vi "test1-TestModuleStatusVI.vi"(8 "error in (no error)":errorcluster, 11 "TestCase in":refnum<class "testcase-CSMManagementAPI.lvclass">) -> (0 "error out":errorcluster, 3 "TestCase out":refnum<class "testcase-CSMManagementAPI.lvclass">)   [LabVIEW 2017, in "testcase-CSMManagementAPI.lvclass"]
uses:
  testcase-CSMManagementAPI.lvclass
  src/user.lib/_NEVSTOP/Communicable State Machine(CSM)/_Support/Typedef/_CSM_MODE.ctl
  src/user.lib/_NEVSTOP/Communicable State Machine(CSM)/AdvanceAPI/CSM - Revert Arguments-Safe String.vi
  src/user.lib/_NEVSTOP/Communicable State Machine(CSM)/_Shared/Trim Single-line Text.vi
  src/user.lib/_NEVSTOP/Communicable State Machine(CSM)/AdvanceAPI/CSM - Make String Arguments Safe.vi
  src/user.lib/_NEVSTOP/Communicable State Machine(CSM)/AdvanceAPI/CSM - Break Down Multiple States String.vi
  src/user.lib/_NEVSTOP/Communicable State Machine(CSM)/AdvanceAPI/CSM - Compact Multiple States.vi
  src/user.lib/_NEVSTOP/Communicable State Machine(CSM)/AdvanceAPI/CSM - Keywords.vi
  <vilib>/addons/_JKI Toolkits/VI Tester/TestCase.llb/TestCase.lvclass
  src/user.lib/_NEVSTOP/Communicable State Machine(CSM)/Communicable State Machine.lvlib
  src/user.lib/_NEVSTOP/Communicable State Machine(CSM)/_Support/Typedef/_CSM_List Module Scope.ctl
  C:/Program Files (x86)/National Instruments/LabVIEW 2017/vi.lib/addons/_JKI Toolkits/VI Tester/TestCase.llb/TestCase.lvclass
panel:
  out "State History":string
  out "LoopCount":i32
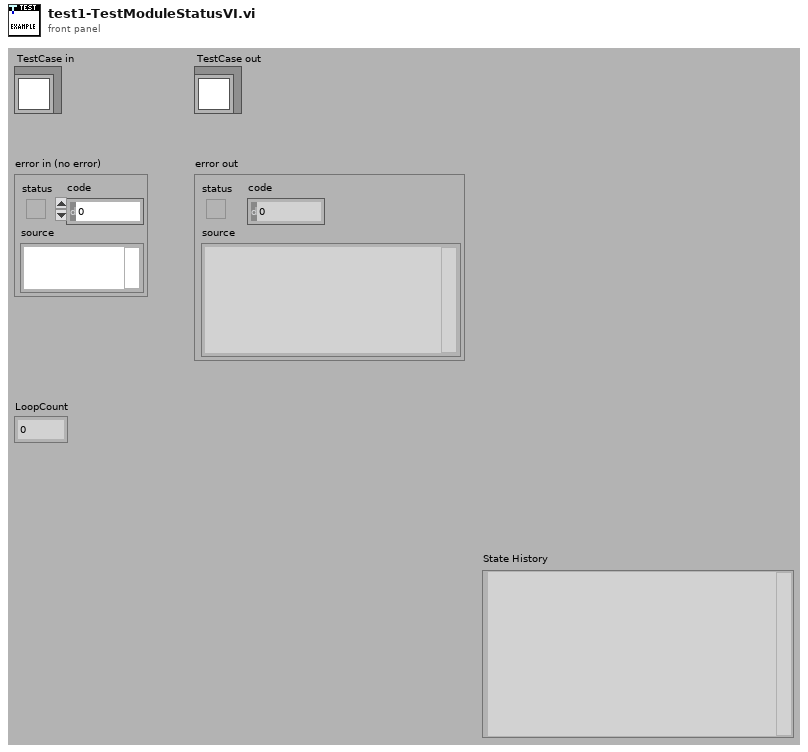
[diagram p1: front panel]
types:
  T1 = typedef "Communicable State Machine.lvlib/_CSM_MODE.ctl" = enum16{"Not Exist", "Stand Alone", "CSM", "Worker", "Worker Agent", "Chain Node", "Chain"}
  T2 = cluster{"CSM Name (Dup)":string, "Mode":T1, "#Nodes":i32}[]
  T3 = typedef "Communicable State Machine.lvlib/_CSM_List Module Scope.ctl" = enum16{"Normal", "System Only", "All"}
  T4 = enum32{"Invalid", "Standard", "Closed", "Hidden", "Minimized", "Maximized"}
  T5 = enum32{"invalid app kind", "Development System", "Run Time System", "Student Edition", "Embedded LabVIEW", "Evaluation", "Custom"}
  T6 = typedef "Communicable State Machine.lvlib/_CSM_Response Source Message.ctl" = cluster{"‘State":string, "’Arguments":string, "’Error":errorcluster}
  T7 = cluster{"Current VI Reference":refnum<vi>, "Close Panel on Exit?":bool}
  T8 = cluster{"Core":cluster{"Current VI Reference":refnum<vi>, "Close Panel on Exit?":bool}, "Your Boolean data":bool, "Your string data":string, "Module Status":cluster{"CSM Name (Dup)":string, "Mode":T1, "#Nodes":i32}}
  T9 = cluster{"CSM Name (Dup)":string, "Mode":T1, "#Nodes":i32}
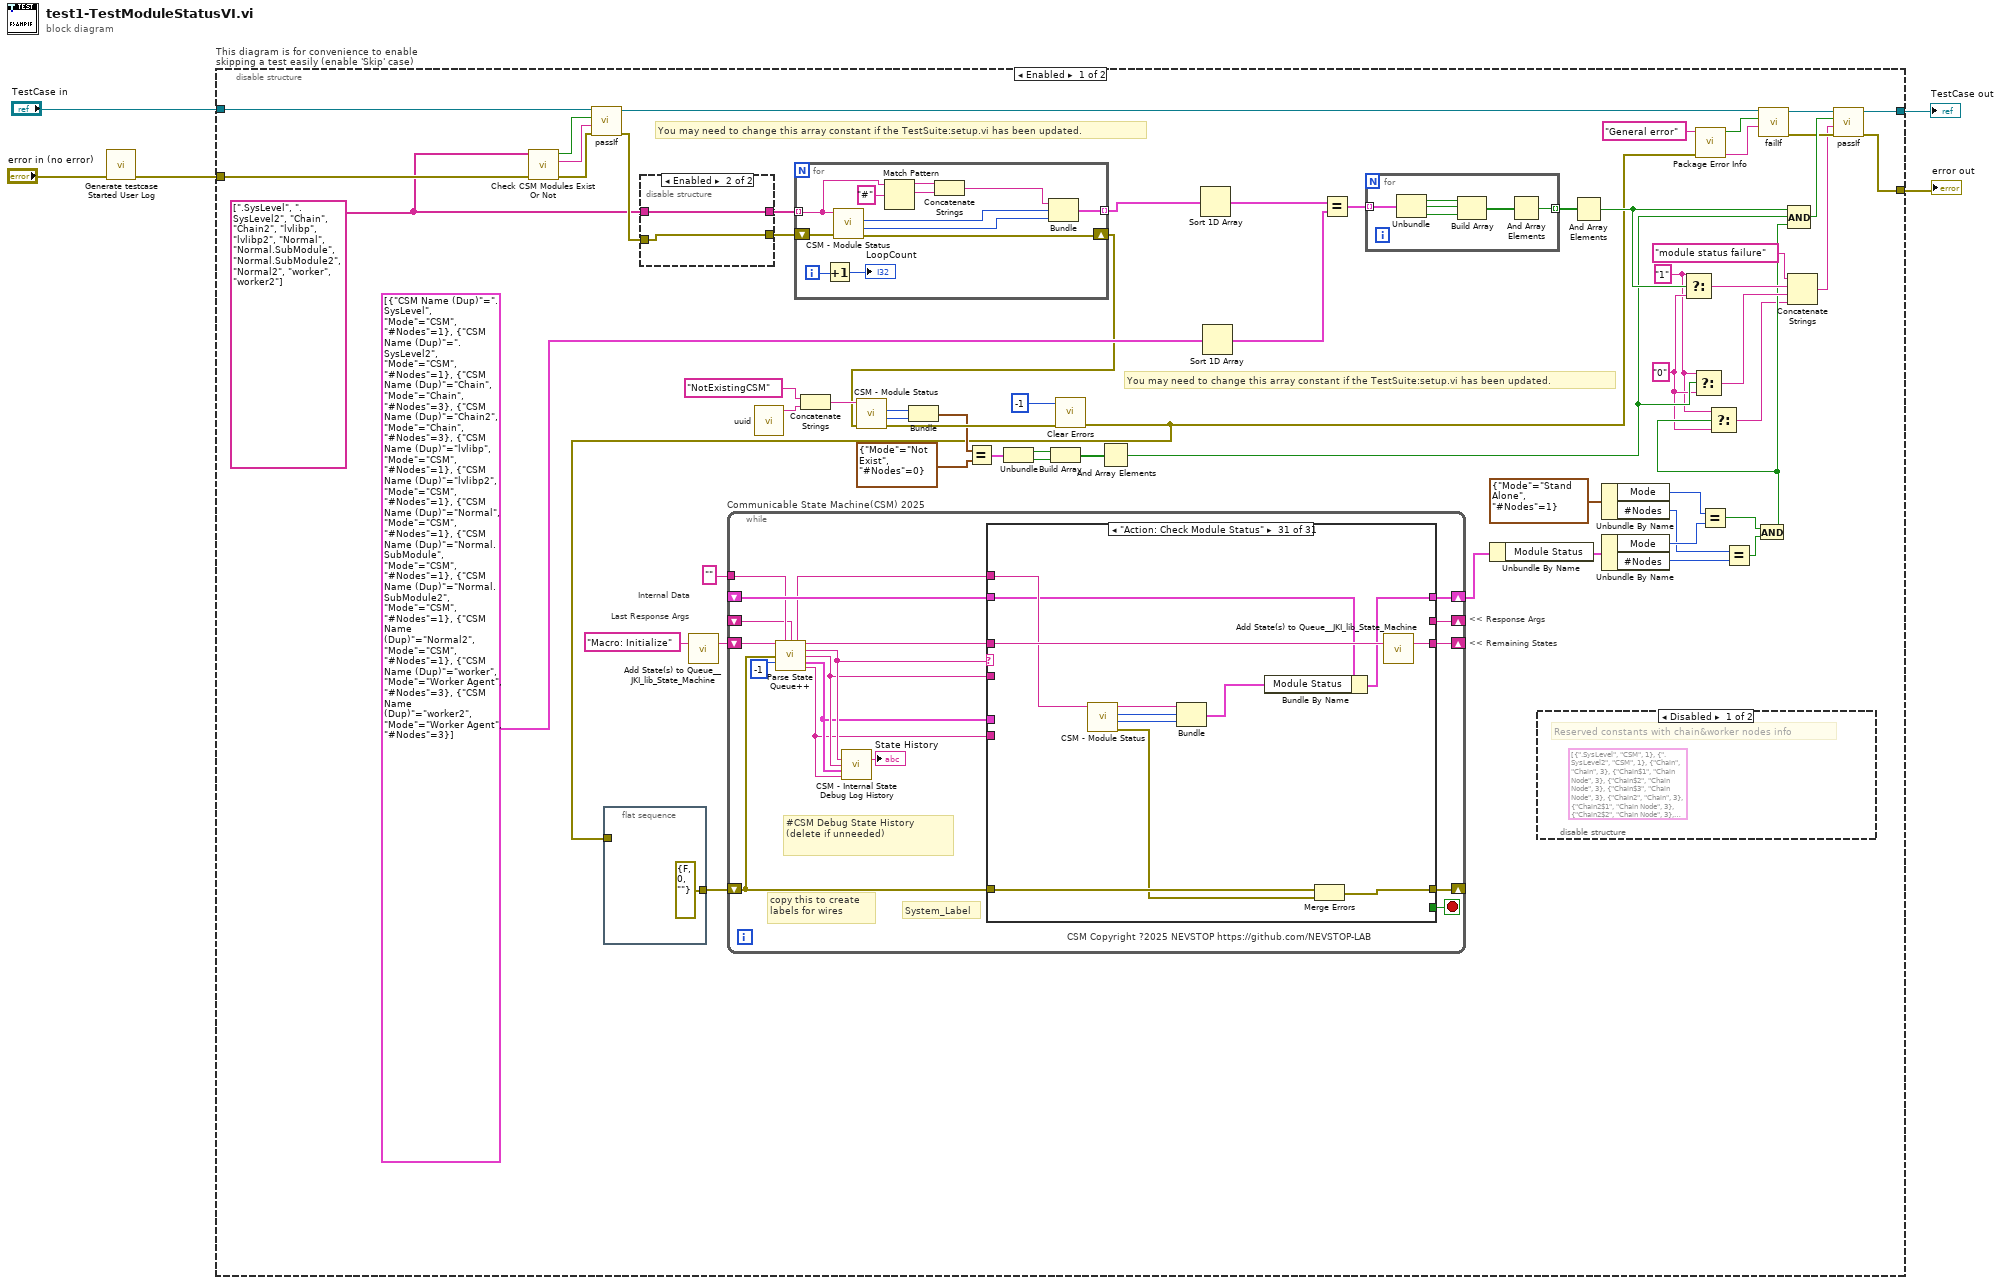
[diagram p0: block diagram]
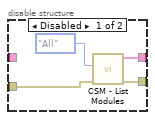
[diagram p3: hidden frame]
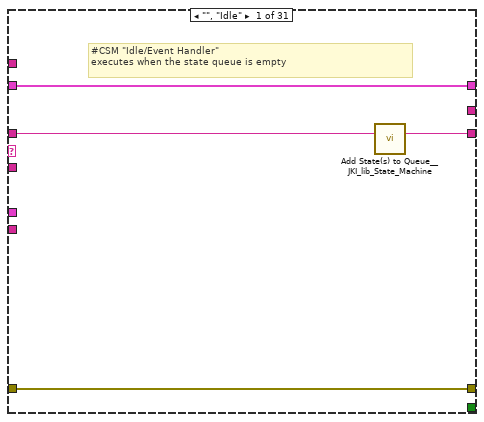
[diagram p4: hidden frame]
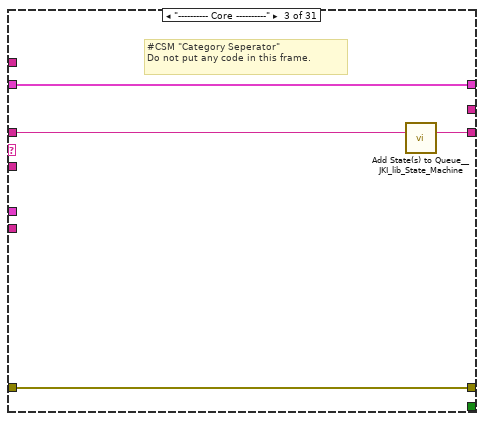
[diagram p6: hidden frame]
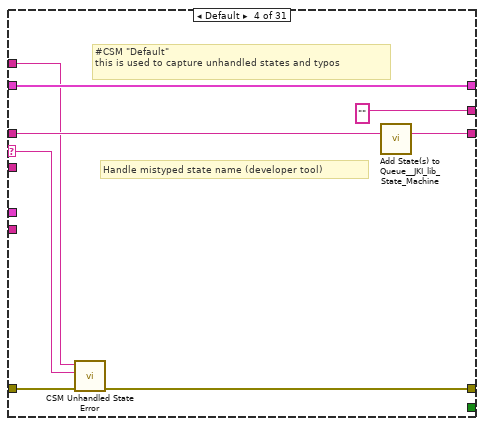
[diagram p7: hidden frame]
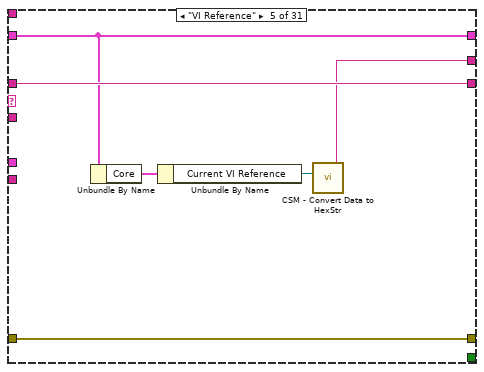
[diagram p8: hidden frame]
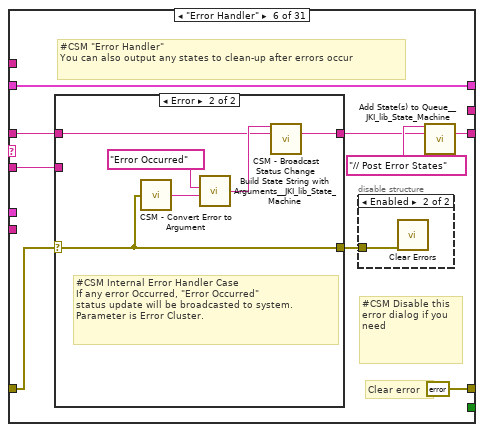
[diagram p9: hidden frame]
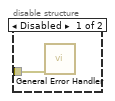
[diagram p10: hidden frame]
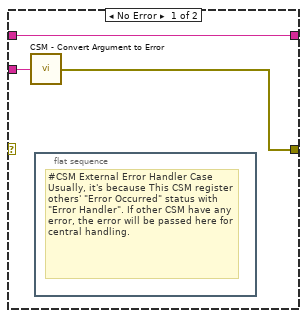
[diagram p11: hidden frame]
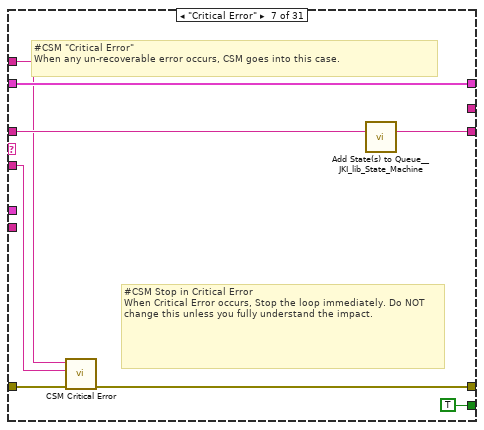
[diagram p12: hidden frame]
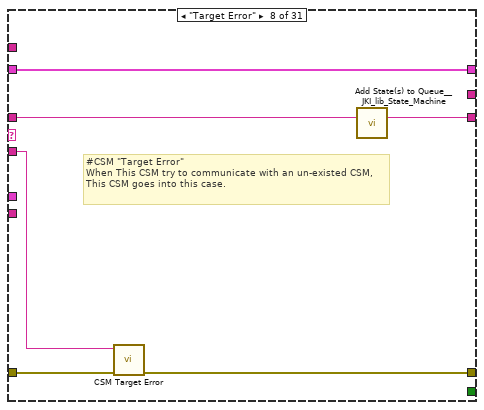
[diagram p13: hidden frame]
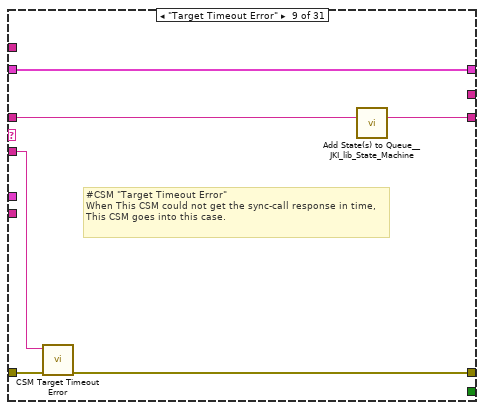
[diagram p14: hidden frame]
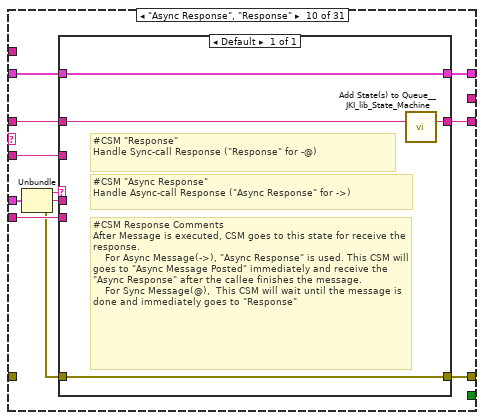
[diagram p15: hidden frame]
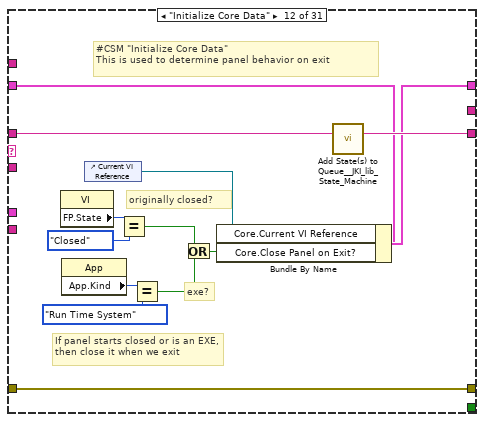
[diagram p17: hidden frame]
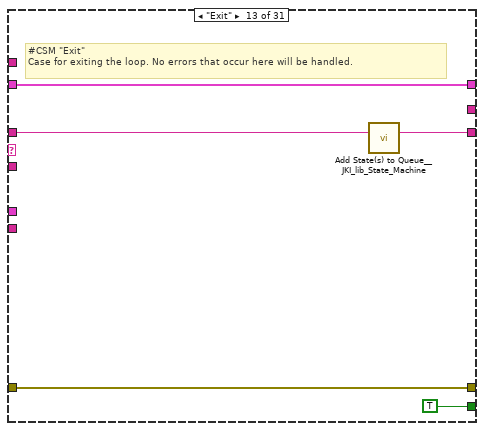
[diagram p18: hidden frame]
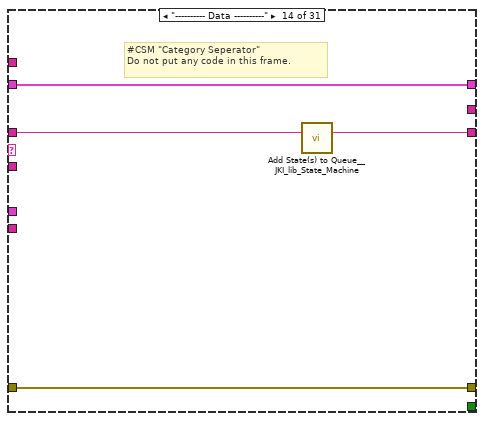
[diagram p19: hidden frame]
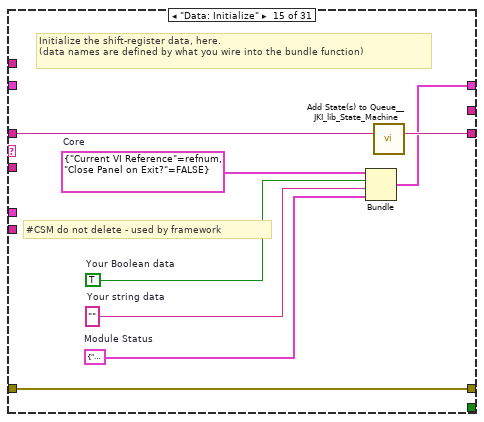
[diagram p20: hidden frame]
diagram:
  n1 = call "Generate testcase Started User Log.vi"("Error In"="error in (no error)") -> ("error out"=w1:errorcluster)  [unwired: 10 in]
  n2 = disable-structure "This diagram is for convenience to enable skipping a test easily (enable 'Skip' case)" shown="Enabled" {
    disable-tunnel: "TestCase in" -> [w27 w384]
    disable-tunnel: [w65 w382] -> w2
    disable-tunnel: [w64 w383] -> w4
    disable-tunnel: w1 -> [w26 w381]
    frame Enabled {
      w12 = "0" ("f")
      w11 = "1"
      w6 = string[] [".SysLevel", ".SysLevel2", "Chain", "Chain2", "lvlibp", "lvlibp2", "Normal", "Normal.SubModule", "Normal.SubModule2", "Normal2", "worker", "worker2"] ("Module Names in All Scope")
      # "You may need to change this array constant if the TestSuite:setup.vi has been updated."
      # "You may need to change this array constant if the TestSuite:setup.vi has been updated."
      # "Last Response Args"
      # "Internal Data"
      # "<< Response Args"
      # "<< Remaining States"
      n3 = call "Check CSM Modules Exist Or Not.vi"("error in"=w26, "CSM names in"=w6) -> ("error out"=w28:errorcluster, "Debug string"=w29:string, "All Modules Exist?"=w30:bool)  [unwired: 7 in]
      n4 = call-dynamic "passIf.vi"("error in (no error)"=w28, "message (\"\")"=w29, "pass"=w30, "TestCase in"=w27) -> ("error out"=w25:errorcluster, "TestCase out"=w22:refnum<class "testcase-CSMManagementAPI.lvclass">)  [unwired: 6 in]
      n5 = flat-sequence {
        tunnel: [errorcluster {"status"=FALSE, "code"=0, "source"=""} ("error out")] -> w63
        tunnel: w7 -> [_]
        frame #0 {
        }
      }
      n6 = disable-structure shown="Enabled" {
        disable-tunnel: [w70 w73] -> w67
        disable-tunnel: [w69 w72] -> w66
        disable-tunnel: w25 -> [w68 w73]
        disable-tunnel: w6 -> [_ w72]
        frame Disabled {
          n7 = call "CSM - List Modules.vi"("Error In"=w68, "Scope (Normal)"=_CSM_List_Module_Scope."All") -> ("error out"=w70:errorcluster, "Module Names"=w69:string[])  [unwired: 8 in]
        }
        frame Enabled {
        }
      }
      n8 = call <vilib>:"Add State(s) to Queue__JKI_lib_State_Machine.vi"("State(s) in (\"\")"="Macro: Initialize" ("Init State(\"Macro: Initialize\")")) -> ("States Out"=w60:string)  [unwired: 14 in]
      n9 = while "Communicable State Machine(CSM) 2025" {
        shift-right: [w93] -> w59
        shift-left: _ -> [w92]
        shift-right: [w96] -> _
        shift-left: w63 -> [w91]
        shift-right: [w95] -> _
        shift-left: w60 -> [w97]
        tunnel: "" ("Name (\"\" to Use UUID)") -> [w89]
        shift-right: [w90] -> _
        shift-left: _ -> [w83]
        stop <- w94 stop-if-true
        # "#CSM Debug State History\n(delete if unneeded)"
        # "copy this to create labels for wires"
        # "System_Label"
        # "CSM Copyright ?2025 NEVSTOP https://github.com/NEVSTOP-LAB"
        n10 = call "Parse State Queue++.vi"("State Queue"=w97, "Name (\"\" to Use UUID)"=w89, "Response Arguments"=w83, "Previous Error"=w91, "Dequeue (1 ms)"=-1 ("Timeout")) -> ("Name Used"=w84:string, "Remaining States"=w98:string, "Current State"=w88:string, "Arguments"=w87:string, "Additional Information"=w86:T6, "Source CSM"=w85:string)  [unwired: 5 in]
        n11 = call "CSM - Internal State Debug Log History.vi"("State"=w88, "Arguments (\"\")"=w87, ">> Response Source Message >>"=w86, "Source (\"\")"=w85) -> ("Debug Log"=→"State History":string)  [unwired: 11 in]
        n12 = case shown="\"Action: Check Module Status\"" w88 {
          selector: w88 -> [_ _ _ w112 _ _ _ _ _ _ _ _ _ _ _ _ _ _ _ _ _ _ _ _ _ _ _ _ _ _ _]
          tunnel: w98 -> [w99 w104 w109 w116 w122 w128 w149 w155 w161 w169 w180 w194 w199 w203 w211 w213 w220 w224 w228 w234 w249 w318 w323 w330 w332 w336 w341 w348 w352 w356 w368]
          tunnel: w87 -> [_ _ _ _ _ w127 w145 w154 w159 w168 _ _ _ _ _ _ _ _ _ w229 w243 _ _ _ _ _ w339 _ _ _ _]
          tunnel: w92 -> [w100 w103 w106 w114 w121 w131 w150 w156 w162 w171 w179 w187 w197 w200 _ w212 w215 w221 w226 w232 w245 w315 w320 w327 w331 w335 w340 w345 w349 w353 w361]
          tunnel: [w101 w105 w107 w110 w123 errorcluster {"status"=FALSE, "code"=0, "source"=""} ("error out") w146 w152 w158 w174 w181 w191 w196 w201 w208 w214 w216 w222 w225 w230 w246 w316 w321 w328 w333 w337 w342 w346 w350 w354 w358] -> w96
          tunnel: w91 -> [w101 w105 w107 w117 w123 w129 w151 w153 w160 _ w181 w191 w196 w201 w208 w214 w217 w222 w225 w231 w247 w316 w321 w328 w333 w337 w342 w346 w350 w354 w366]
          tunnel: [w102 w104 w108 w115 w122 w124 w148 w157 w163 w170 w180 w193 w198 w202 w210 w213 w219 w223 w227 w233 w248 w317 w322 w329 w332 w336 w341 w347 w351 w355 w367] -> w95
          tunnel: [_ _ _ _ _ _ TRUE _ _ _ _ _ TRUE _ _ _ _ _ _ _ _ _ _ _ _ _ _ _ _ _ _] -> w94
          tunnel: [w100 w103 w106 w114 w121 w131 w150 w156 w162 w172 w179 w192 w197 w200 w209 w212 w215 w221 w226 w232 w245 w315 w320 w327 w331 w335 w340 w345 w349 w353 w360] -> w93
          tunnel: w85 -> [_ _ _ _ _ _ _ _ _ w166 _ _ _ _ _ _ _ _ _ _ _ _ _ _ _ _ _ _ _ _ _]
          tunnel: w86 -> [_ _ _ _ _ _ _ _ _ w173 _ _ _ _ _ _ _ _ _ _ _ _ _ _ _ _ _ _ _ _ _]
          tunnel: [_ _ _ "" w118 _ _ _ _ _ _ _ _ _ _ _ _ _ _ _ _ _ _ _ _ "API1 Response" w338 _ _ _ _] -> w90
          tunnel: w84 -> [_ _ _ w111 _ _ w144 _ _ _ _ _ _ _ _ _ _ _ _ _ _ _ _ _ _ _ _ _ _ _ w365]
          frame "", "Idle" {
            # "#CSM \"Idle/Event Handler\"\nexecutes when the state queue is empty"
            n13 = call <vilib>:"Add State(s) to Queue__JKI_lib_State_Machine.vi"("State(s) in (\"\")"=w99) -> ("States Out"=w102:string)  [unwired: 14 in]
          }
          frame "CSM Documentation" {
            # "#CSM README FIRST\n\nCommunicable State Machine(CSM) is a LabVIEW application framework that builds upon JKI State Machine(JKISM). It follows the pattern of JKISM and extends the keywords to describe message communication between modules, including concepts such as Sync-Message, Async-Message, Subscription/Unsubscription of status - essential elements for creating reusable code modules. For more information, please visit the CSM wiki: https://nevstop-lab.github.io/CSM-Wiki/\n\nFor instructions on JKI State Machine, visit: http://jki.net/state-machine/\nFor information about CSM, visit: https://github.com/NEVSTOP-LAB"
            # "#CSM \"Documentation\"\nCase for holding CSM Documenation"
          }
          frame "---------- Core ----------" {
            # "#CSM \"Category Seperator\"\nDo not put any code in this frame."
            n14 = call <vilib>:"Add State(s) to Queue__JKI_lib_State_Machine.vi"("State(s) in (\"\")"=w109) -> ("States Out"=w108:string)  [unwired: 14 in]
          }
          frame Default {
            # "#CSM \"Default\"\nthis is used to capture unhandled states and typos"
            # "Handle mistyped state name (developer tool)"
            n15 = call "CSM Unhandled State Error.vi"("error in (no error)"=w117, "Undefined State"=w112, "CSM Name"=w111) -> ("error out"=w110:errorcluster)  [unwired: 8 in]
            n16 = call <vilib>:"Add State(s) to Queue__JKI_lib_State_Machine.vi"("State(s) in (\"\")"=w116) -> ("States Out"=w115:string)  [unwired: 14 in]
          }
          frame "VI Reference" {
            n17 = Unbundle By Name(w121) -> ("Core"=w120:T7)
            n18 = Unbundle By Name(w120) -> ("Current VI Reference"=w119:refnum<vi>)
            n19 = call "CSM - Convert Data to HexStr.vi"("Variant"=w119) -> ("HEX String (0-9,A-F)"=w118:string)  [unwired: 8 in]
          }
          frame "Error Handler" {
            # "#CSM Disable this error dialog if you need"
            # "#CSM \"Error Handler\"\nYou can also output any states to clean-up after errors occur"
            # "Clear error"
            n20 = case shown="Error" w129 {
              selector: w129 -> [_ w138]
              tunnel: [w137 w140] -> w125
              tunnel: w128 -> [w137 w139]
              tunnel: w127 -> [w136 _]
              tunnel: [w135 w138] -> w130
              frame No Error {
                n21 = call "CSM - Convert Argument to Error.vi"("Argument"=w136) -> ("Error"=w135:errorcluster)  [unwired: 4 in]
                n22 = flat-sequence {
                  frame #0 {
                    # "#CSM External Error Handler Case\nUsually, it's because This CSM register others' \"Error Occurred\" status with \"Error Handler\". If other CSM have any error, the error will be passed here for central handling."
                  }
                }
              }
              frame Error {
                # "#CSM Internal Error Handler Case \nIf any error Occurred, \"Error Occurred\" \nstatus update will be broadcasted to system.\nParameter is Error Cluster."
                n23 = call "CSM - Convert Error to Argument.vi"("Error"=w138) -> ("Argument"=w142:string)  [unwired: 4 in]
                n24 = call <vilib>:"Build State String with Arguments__JKI_lib_State_Machine.vi"("Arguments (\"\")"=w142, "State"="Error Occurred" ("Status with Arguments")) -> ("State with Arguments"=w141:string)  [unwired: 4 in]
                n25 = call "CSM - Broadcast Status Change.vi"("Status With Arguments"=w141, "State Queue"=w139) -> ("Remaining States"=w140:string)  [unwired: 13 in]
              }
            }
            n26 = disable-structure shown="Enabled" {
              disable-tunnel: w130 -> [w133 w134]
              frame Disabled {
                n27 = call <vilib>:"General Error Handler.vi"("error in (no error)"=w133) -> ()  [unwired: 10 in, 5 out]
              }
              frame Enabled {
                n28 = call <vilib>:"Clear Errors.vi"("error in (no error)"=w134) -> ()  [unwired: 5 in, 2 out]
              }
            }
            n29 = call <vilib>:"Add State(s) to Queue__JKI_lib_State_Machine.vi"("State(s) in Front (\"\")"="// Post Error States", "State(s) in (\"\")"=w125) -> ("States Out"=w124:string)  [unwired: 13 in]
          }
          frame "Critical Error" {
            # "#CSM Stop in Critical Error\nWhen Critical Error occurs, Stop the loop immediately. Do NOT change this unless you fully understand the impact."
            # "#CSM \"Critical Error\"\nWhen any un-recoverable error occurs, CSM goes into this case."
            n30 = call "CSM Critical Error.vi"("error in (no error)"=w151, "Arugments (As Reason)"=w145, "CSM Name"=w144) -> ("error out"=w146:errorcluster)  [unwired: 8 in]
            n31 = call <vilib>:"Add State(s) to Queue__JKI_lib_State_Machine.vi"("State(s) in (\"\")"=w149) -> ("States Out"=w148:string)  [unwired: 14 in]
          }
          frame "Target Error" {
            # "#CSM \"Target Error\"\nWhen This CSM try to communicate with an un-existed CSM, This CSM goes into this case."
            n32 = call "CSM Target Error.vi"("error in (no error)"=w153, "Arguments (As CSM Name)"=w154) -> ("error out"=w152:errorcluster)  [unwired: 9 in]
            n33 = call <vilib>:"Add State(s) to Queue__JKI_lib_State_Machine.vi"("State(s) in (\"\")"=w155) -> ("States Out"=w157:string)  [unwired: 14 in]
          }
          frame "Target Timeout Error" {
            # "#CSM \"Target Timeout Error\"\nWhen This CSM could not get the sync-call response in time, This CSM goes into this case."
            n34 = call "CSM Target Timeout Error.vi"("error in (no error)"=w160, "Arguments (As CSM Name)"=w159) -> ("error out"=w158:errorcluster)  [unwired: 9 in]
            n35 = call <vilib>:"Add State(s) to Queue__JKI_lib_State_Machine.vi"("State(s) in (\"\")"=w161) -> ("States Out"=w163:string)  [unwired: 14 in]
          }
          frame "Async Response", "Response" {
            n36 = Unbundle(w173) -> ("‘State"=w167:string, "’Arguments"=w165:string, "’Error"=w164:errorcluster)
            n37 = case shown="Default" w167 {
              tunnel: [w178] -> w174
              tunnel: w164 -> [w178]
              tunnel: [w177] -> w172
              tunnel: w171 -> [w177]
              tunnel: [w175] -> w170
              tunnel: w169 -> [w176]
              tunnel: w168 -> [_]
              tunnel: w166 -> [_]
              tunnel: w165 -> [_]
              frame Default {
                # "#CSM Response Comments\nAfter Message is executed, CSM goes to this state for receive the response.\n    For Async Message(->), \"Async Response\" is used. This CSM will goes to \"Async Message Posted\" immediately and receive the \"Async Response\" after the callee finishes the message.\n    For Sync Message(@),  This CSM will wait until the message is done and immediately goes to \"Response\""
                # "#CSM \"Async Response\"\nHandle Async-call Response (\"Async Response\" for ->)"
                # "#CSM \"Response\"\nHandle Sync-call Response (\"Response\" for -@)"
                n38 = call <vilib>:"Add State(s) to Queue__JKI_lib_State_Machine.vi"("State(s) in (\"\")"=w176) -> ("States Out"=w175:string)  [unwired: 14 in]
              }
            }
          }
          frame "Async Message Posted" {
            # "#CSM \"Async Message Posted\"\nAfter Async Message is posted (-> or ->| ), CSM goes to this state for post-action.\nYou can use Argument - State to tell which Async Message is called."
          }
          frame "Initialize Core Data" {
            # "#CSM \"Initialize Core Data\"\nThis is used to determine panel behavior on exit"
            # "originally closed?"
            # "exe?"
            # "If panel starts closed or is an EXE, then close it when we exit"
            n39 = property class="VI"() -> ("FP.State"=w184:T4)  [unwired: 2 in, 2 out]
            n40 = property class="App"() -> ("App.Kind"=w190:T5)  [unwired: 2 in, 2 out]
            n41 = control-ref of="Current VI Reference"() -> (w185:refnum<vi>)
            n42 = Equal?(x=w184, y=T4."Closed" ("Front Panel Window:State")) -> (x = y?=w182:bool)
            n43 = Equal?(x=w190, y=T5."Run Time System" ("Application:Kind")) -> (x = y?=w188:bool)
            n44 = Or(x=w182, y=w188) -> (x .or. y?=w186:bool)
            n45 = Bundle By Name(cluster=w187, "Core.Current VI Reference"=w185, "Core.Close Panel on Exit?"=w186) -> (w192:T8)
            n46 = call <vilib>:"Add State(s) to Queue__JKI_lib_State_Machine.vi"("State(s) in (\"\")"=w194) -> ("States Out"=w193:string)  [unwired: 14 in]
          }
          frame "Exit" {
            # "#CSM \"Exit\"\nCase for exiting the loop. No errors that occur here will be handled."
            n47 = call <vilib>:"Add State(s) to Queue__JKI_lib_State_Machine.vi"("State(s) in (\"\")"=w199) -> ("States Out"=w198:string)  [unwired: 14 in]
          }
          frame "---------- Data ----------" {
            # "#CSM \"Category Seperator\"\nDo not put any code in this frame."
            n48 = call <vilib>:"Add State(s) to Queue__JKI_lib_State_Machine.vi"("State(s) in (\"\")"=w203) -> ("States Out"=w202:string)  [unwired: 14 in]
          }
          frame "Data: Initialize" {
            w204 = T9 {"CSM Name (Dup)"="", "Mode"=enum."Not Exist", "#Nodes"=0}  # Module Status
            w205 = T7 {"Current VI Reference"=refnum, "Close Panel on Exit?"=FALSE}  # Core
            w207 = TRUE  # Your Boolean data
            w206 = ""  # Your string data
            # "#CSM do not delete - used by framework"
            # "Initialize the shift-register data, here.\n(data names are defined by what you wire into the bundle function)"
            n49 = Bundle("Core"=w205, "Your Boolean data"=w207, "Your string data"=w206, "Module Status"=w204) -> (w209:T8)  [unwired: 1 in]
            n50 = call <vilib>:"Add State(s) to Queue__JKI_lib_State_Machine.vi"("State(s) in (\"\")"=w211) -> ("States Out"=w210:string)  [unwired: 14 in]
          }
          frame "Data: Update Indicators" {
          }
          frame "Data: Cleanup" {
            # "Cleanup any data and references, here.\n(this is called automatically, by the Macro: Exit)"
            n51 = Unbundle By Name(w215) -> ("Core.Current VI Reference"=w218:refnum<vi>)
            n52 = Close Reference(reference=w218, error in (no error)=w217) -> (error out=w216:errorcluster)
            n53 = call <vilib>:"Add State(s) to Queue__JKI_lib_State_Machine.vi"("State(s) in (\"\")"=w220) -> ("States Out"=w219:string)  [unwired: 14 in]
          }
          frame "---------- UI ----------" {
            # "#CSM \"Category Seperator\"\nDo not put any code in this frame."
            n54 = call <vilib>:"Add State(s) to Queue__JKI_lib_State_Machine.vi"("State(s) in (\"\")"=w224) -> ("States Out"=w223:string)  [unwired: 14 in]
          }
          frame "UI: Initialize" {
            # "#CSM \"UI: Initialize\"\nInitialize the User Interface, here.\n(this is called automatically, by the Macro: Init)"
            n55 = call <vilib>:"Add State(s) to Queue__JKI_lib_State_Machine.vi"("State(s) in (\"\")"=w228) -> ("States Out"=w227:string)  [unwired: 14 in]
          }
          frame "UI: Cursor Set" {
            # "#CSM \"UI: Cursor Set\"\nSet and Unset Cursor Busy.\n(Usage: \"UI: Cursor Set >> Busy|Idle\")"
            # "Argument"
            n56 = disable-structure shown="TARGET_TYPE!=Windows" {
              disable-tunnel: w231 -> [w237 w242]
              disable-tunnel: [w236 w242] -> w230
              disable-tunnel: w229 -> [w235 _]
              frame condition #0 (active) {
                n57 = case shown="\"Idle\", Default" w235 {
                  tunnel: w237 -> [w239 w241]
                  tunnel: [w238 w240] -> w236
                  frame "Idle", Default {
                    n58 = call <vilib>:"Unset Busy.vi"("error in (no error)"=w239) -> ("error out"=w238:errorcluster)  [unwired: 10 in]
                  }
                  frame "Busy" {
                    n59 = call <vilib>:"Set Busy.vi"("error in (no error)"=w241) -> ("error out"=w240:errorcluster)  [unwired: 9 in, 1 out]
                  }
                }
              }
              frame condition #1 {
              }
            }
            n60 = call <vilib>:"Add State(s) to Queue__JKI_lib_State_Machine.vi"("State(s) in (\"\")"=w234) -> ("States Out"=w233:string)  [unwired: 14 in]
          }
          frame "UI: Front Panel State" {
            # "#CSM \"UI: Front Panel State\"\nSet Front Panel Open or Closed\n(Usage: \"UI: Front Panel State >> Open|Close\")"
            # "Argument"
            n61 = Unbundle By Name(w245) -> ("Core.Current VI Reference"=w244:refnum<vi>)
            n62 = call <vilib>:"Add State(s) to Queue__JKI_lib_State_Machine.vi"("State(s) in (\"\")"=w249) -> ("States Out"=w248:string)  [unwired: 14 in]
            n63 = case shown="\"Close\", \"Closed\"" w243 {
              tunnel: w247 -> [w255 w270 w281 w294 w307]
              tunnel: [w257 w271 w283 w296 w309] -> w246
              tunnel: w244 -> [w256 w268 w282 w295 w308]
              frame "Open", "Standard", Default {
                w250 = T4."Standard" ("State")
                n64 = property class="VI"(reference=w256, error in=w255) -> (reference out=w253:refnum<vi>, error out=w254:errorcluster, "FP.State"=w252:T4)
                n65 = Not Equal?(x=w252, y=w250) -> (x != y?=w251:bool)
                n66 = case shown="True" w251 {
                  tunnel: [w261 w263] -> w257
                  tunnel: w254 -> [w260 w263]
                  tunnel: w253 -> [w259 _]
                  tunnel: w250 -> [w258 _]
                  frame True {
                    n67 = invoke class="VI" method="FP.Open"(reference=w259, error in=w260, "Activate"=TRUE, "State"=w258) -> (error out=w261:errorcluster)  [unwired: 1 in, 4 out]
                  }
                  frame False {
                  }
                }
              }
              frame "Close", "Closed" {
                n68 = property class="VI"(reference=w268, error in=w270) -> (reference out=w267:refnum<vi>, error out=w269:errorcluster, "FP.State"=w265:T4)
                n69 = Not Equal?(x=w265, y=T4."Closed" ("Front Panel Window:State")) -> (x != y?=w264:bool)
                n70 = case shown="False" w264 {
                  tunnel: [w272 w275] -> w271
                  tunnel: w269 -> [w272 w274]
                  tunnel: w267 -> [_ w273]
                  frame False {
                  }
                  frame True {
                    n71 = invoke class="VI" method="FP.Close"(reference=w273, error in=w274) -> (error out=w275:errorcluster)  [unwired: 1 in, 2 out]
                  }
                }
              }
              frame "Hidden", "Hide" {
                w276 = T4."Hidden" ("State")
                n72 = property class="VI"(reference=w282, error in=w281) -> (reference out=w279:refnum<vi>, error out=w280:errorcluster, "FP.State"=w278:T4)
                n73 = Not Equal?(x=w278, y=w276) -> (x != y?=w277:bool)
                n74 = case shown="True" w277 {
                  tunnel: [w287 w288] -> w283
                  tunnel: w280 -> [w286 w288]
                  tunnel: w279 -> [w285 _]
                  tunnel: w276 -> [w284 _]
                  frame True {
                    n75 = invoke class="VI" method="FP.Open"(reference=w285, error in=w286, "State"=w284) -> (error out=w287:errorcluster)  [unwired: 2 in, 4 out]
                  }
                  frame False {
                  }
                }
              }
              frame "Minimize", "Minimized" {
                w289 = T4."Minimized" ("State")
                n76 = property class="VI"(reference=w295, error in=w294) -> (reference out=w292:refnum<vi>, error out=w293:errorcluster, "FP.State"=w291:T4)
                n77 = Not Equal?(x=w291, y=w289) -> (x != y?=w290:bool)
                n78 = case shown="True" w290 {
                  tunnel: [w300 w301] -> w296
                  tunnel: w293 -> [w299 w301]
                  tunnel: w292 -> [w298 _]
                  tunnel: w289 -> [w297 _]
                  frame True {
                    n79 = invoke class="VI" method="FP.Open"(reference=w298, error in=w299, "State"=w297) -> (error out=w300:errorcluster)  [unwired: 2 in, 4 out]
                  }
                  frame False {
                  }
                }
              }
              frame "Maximize", "Maximized" {
                w302 = T4."Maximized" ("State")
                n80 = property class="VI"(reference=w308, error in=w307) -> (reference out=w305:refnum<vi>, error out=w306:errorcluster, "FP.State"=w304:T4)
                n81 = Not Equal?(x=w304, y=w302) -> (x != y?=w303:bool)
                n82 = case shown="True" w303 {
                  tunnel: [w313 w314] -> w309
                  tunnel: w306 -> [w312 w314]
                  tunnel: w305 -> [w311 _]
                  tunnel: w302 -> [w310 _]
                  frame True {
                    n83 = invoke class="VI" method="FP.Open"(reference=w311, error in=w312, "State"=w310) -> (error out=w313:errorcluster)  [unwired: 2 in, 4 out]
                  }
                  frame False {
                  }
                }
              }
            }
          }
          frame "---------- Macro ----------" {
            # "#CSM \"Category Seperator\"\nDo not put any code in this frame."
            n84 = call <vilib>:"Add State(s) to Queue__JKI_lib_State_Machine.vi"("State(s) in (\"\")"=w318) -> ("States Out"=w317:string)  [unwired: 14 in]
          }
          frame "Macro: Initialize" {
            # "#CSM \"Macro: Initialize\"\nInitialization Macro (This is called once, when the VI starts)"
            n85 = call <vilib>:"Add State(s) to Queue__JKI_lib_State_Machine.vi"("State(s) in Front (\"\")"="Data: Initialize\nInitialize Core Data\nData: Update Indicators\nAction: Check Module Status\nMacro: Exit", "State(s) in (\"\")"=w323) -> ("States Out"=w322:string)  [unwired: 13 in]
          }
          frame "Macro: Exit" {
            # "#CSM \"Macro: Exit\"\nExit Macro (This is called once, when the VI exits)"
            n86 = call <vilib>:"Add State(s) to Queue__JKI_lib_State_Machine.vi"("State(s) in Front (\"\")"="//Exit Sub-Modules ", "State(s) at Back (\"\")"="Data: Cleanup\nExit") -> ("States Out"=w325:string)  [unwired: 13 in]
            n87 = call <vilib>:"Add State(s) to Queue__JKI_lib_State_Machine.vi"("State(s) in Front (\"\")"=w325, "State(s) in (\"\")"=w330) -> ("States Out"=w329:string)  [unwired: 13 in]
          }
          frame "---------- API ----------" {
            # "#CSM \"Category Seperator\"\nDo not put any code in this frame."
          }
          frame "API: API1" {
            # "#CSM API Example\nCopy/Rename this case for your own API"
            # "#CSM Response\nConnect this to return the response of your API"
            # "#CSM >> Msg/Rep's CSM >>\nIf you need to tell who triggered this state , use this string. If it's this case itself, this string is \"\"."
            # "#CSM >> Arguments >>\nDeal with the parameter if any"
          }
          frame "API: API2" {
            # "#CSM API Example\nCopy/Rename this case for your own API"
            # "unpack Hex String  to Variant\nif complex parameter is needed."
            n88 = call "CSM - Convert HexStr to Data.vi"("HEX String"=w339) -> ()  [unwired: 7 in, 2 out]
            n89 = disable-structure shown="Disabled" {
              disable-tunnel: [w343 "API2 Response"] -> w338
              frame Disabled {
                # "pack variant to hexstr \nif complex response is needed."
                # "complex Response"
                n90 = call "CSM - Convert Data to HexStr.vi"() -> ("HEX String (0-9,A-F)"=w343:string)  [unwired: 9 in]
              }
              frame Enabled {
              }
            }
          }
          frame "---------- Action ----------" {
            # "#CSM \"Category Seperator\"\nDo not put any code in this frame."
            n91 = call <vilib>:"Add State(s) to Queue__JKI_lib_State_Machine.vi"("State(s) in (\"\")"=w348) -> ("States Out"=w347:string)  [unwired: 14 in]
          }
          frame "Action: action1" {
            # "#CSM \"Internal State\"\nThis category is used for holding internal states"
            n92 = call <vilib>:"Add State(s) to Queue__JKI_lib_State_Machine.vi"("State(s) in (\"\")"=w352) -> ("States Out"=w351:string)  [unwired: 14 in]
          }
          frame "Action: action2" {
            # "#CSM \"Internal State\"\nThis category is used for holding internal states"
            n93 = call <vilib>:"Add State(s) to Queue__JKI_lib_State_Machine.vi"("State(s) in (\"\")"=w356) -> ("States Out"=w355:string)  [unwired: 14 in]
          }
          frame "Action: Check Module Status" {
            n94 = call "CSM - Module Status.vi"("CSM Name"=w365) -> ("error out"=w357:errorcluster, "#Nodes"=w362:i32, "Mode"=w363:T1, "CSM Name (Dup)"=w364:string)  [unwired: 6 in, 1 out]
            n95 = Bundle("CSM Name (Dup)"=w364, "Mode"=w363, "#Nodes"=w362) -> (w359:T9)  [unwired: 1 in]
            n96 = Bundle By Name(cluster=w361, "Module Status"=w359) -> (w360:T8)
            n97 = Merge Errors(w366, w357) -> (w358:errorcluster)
            n98 = call <vilib>:"Add State(s) to Queue__JKI_lib_State_Machine.vi"("State(s) in (\"\")"=w368) -> ("States Out"=w367:string)  [unwired: 14 in]
          }
        }
      }
      n99 = call "uuid.vi"() -> ("UUID"=w53:string)  [unwired: 11 in]
      n100 = for {
        tunnel: w66 -> [w372] mode=indexing
        shift-right: [w379] -> w8
        shift-left: w67 -> [w380]
        tunnel: [w374] -> w51 mode=indexing
        i -> [w378]
        n101 = Increment(x=w378) -> (x+1=→"LoopCount":i32)
        n102 = call "CSM - Module Status.vi"("Error In"=w380, "CSM Name"=w372) -> ("error out"=w379:errorcluster, "#Nodes"=w375:i32, "Mode"=w376:T1)  [unwired: 5 in, 2 out]
        n103 = Match Pattern(string=w372, regular expression="#") -> (before substring=w371:string, match substring=w370:string)  [unwired: 1 in, 2 out]
        n104 = Concatenate Strings(w371, w370) -> (w369:string)
        n105 = Bundle(w369, "Mode"=w376, "#Nodes"=w375) -> (w374:cluster{string, "Mode":T1, "#Nodes":i32})  [unwired: 1 in]
      }
      n106 = Concatenate Strings("NotExistingCSM" ("CSM Name"), w53) -> (w52:string)
      n107 = call "CSM - Module Status.vi"("Error In"=w8, "CSM Name"=w52) -> ("error out"=w56:errorcluster, "#Nodes"=w57:i32, "Mode"=w58:T1)  [unwired: 5 in, 2 out]
      n108 = Bundle("Mode"=w58, "#Nodes"=w57) -> (w45:cluster{"Mode":T1, "#Nodes":i32})  [unwired: 1 in]
      n109 = Equal?(x=w45, y=cluster{"Mode":T1, "#Nodes":i32} {"Mode"=enum."Not Exist", "#Nodes"=0} ("Module Status")) -> (x = y?=w43:cluster{"Mode":bool, "#Nodes":bool})
      n110 = Unbundle(w43) -> ("Mode"=w42:bool, "#Nodes"=w41:bool)
      n111 = Build Array(w42, w41) -> (w40:bool[])
      n112 = call <vilib>:"Clear Errors.vi"("error in (no error)"=w56, "specific error code to clear (0: all)"=-1) -> ("error out"=w7:errorcluster)  [unwired: 4 in, 1 out]
      n113 = And Array Elements(Boolean array=w40) -> (logical AND=w15:bool)
      n114 = Sort 1D Array(array=w51) -> (sorted array=w49:cluster{string, "Mode":T1, "#Nodes":i32}[])
      n115 = Sort 1D Array(array=T2 [{"CSM Name (Dup)"=".SysLevel", "Mode"=enum."CSM", "#Nodes"=1}, {"CSM Name (Dup)"=".SysLevel2", "Mode"=enum."CSM", "#Nodes"=1}, {"CSM Name (Dup)"="Chain", "Mode"=enum."Chain", "#Nodes"=3}, {"CSM Name (Dup)"="Chain2", "Mode"=enum."Chain", "#Nodes"=3}, {"CSM Name (Dup)"="lvlibp", "Mode"=enum."CSM", "#Nodes"=1}, {"CSM Name (Dup)"="lvlibp2", "Mode"=enum."CSM", "#Nodes"=1}, {"CSM Name (Dup)"="Normal", "Mode"=enum."CSM", "#Nodes"=1}, {"CSM Name (Dup)"="Normal.SubModule", "Mode"=enum."CSM", "#Nodes"=1}, {"CSM Name (Dup)"="Normal.SubModule2", "Mode"=enum."CSM", "#Nodes"=1}, {"CSM Name (Dup)"="Normal2", "Mode"=enum."CSM", "#Nodes"=1}, {"CSM Name (Dup)"="worker", "Mode"=enum."Worker Agent", "#Nodes"=3}, {"CSM Name (Dup)"="worker2", "Mode"=enum."Worker Agent", "#Nodes"=3}] ("Module Status Array 2")) -> (sorted array=w48:T2)
      n116 = Equal?(x=w49, y=w48) -> (x = y?=w47:cluster{bool, "Mode":bool, "#Nodes":bool}[])
      n117 = for {
        tunnel: w47 -> [w80] mode=indexing
        tunnel: [w75] -> w46 mode=indexing
        n118 = Unbundle(w80) -> (w79:bool, "Mode"=w78:bool, "#Nodes"=w77:bool)
        n119 = Build Array(w79, w78, w77) -> (w76:bool[])
        n120 = And Array Elements(Boolean array=w76) -> (logical AND=w75:bool)
      }
      n121 = Unbundle By Name(w59) -> ("Module Status"=w39:T9)
      n122 = disable-structure shown="Disabled" {
        frame Disabled {
          (unwired) T2 [{"CSM Name (Dup)"=".SysLevel", "Mode"=enum."CSM", "#Nodes"=1}, {"CSM Name (Dup)"=".SysLevel2", "Mode"=enum."CSM", "#Nodes"=1}, {"CSM Name (Dup)"="Chain", "Mode"=enum."Chain", "#Nodes"=3}, {"CSM Name (Dup)"="Chain$1", "Mode"=enum."Chain Node", "#Nodes"=3}, {"CSM Name (Dup)"="Chain$2", "Mode"=enum."Chain Node", "#Nodes"=3}, {"CSM Name (Dup)"="Chain$3", "Mode"=enum."Chain Node", "#Nodes"=3}, {"CSM Name (Dup)"="Chain2", "Mode"=enum."Chain", "#Nodes"=3}, {"CSM Name (Dup)"="Chain2$1", "Mode"=enum."Chain Node", "#Nodes"=3}, {"CSM Name (Dup)"="Chain2$2", "Mode"=enum."Chain Node", "#Nodes"=3}, {"CSM Name (Dup)"="Chain2$3", "Mode"=enum."Chain Node", "#Nodes"=3}, {"CSM Name (Dup)"="lvlibp", "Mode"=enum."CSM", "#Nodes"=1}, {"CSM Name (Dup)"="lvlibp2", "Mode"=enum."CSM", "#Nodes"=1}, {"CSM Name (Dup)"="Normal", "Mode"=enum."CSM", "#Nodes"=1}, {"CSM Name (Dup)"="Normal.SubModule", "Mode"=enum."CSM", "#Nodes"=1}, {"CSM Name (Dup)"="Normal.SubModule2", "Mode"=enum."CSM", "#Nodes"=1}, {"CSM Name (Dup)"="Normal2", "Mode"=enum."CSM", "#Nodes"=1}, {"CSM Name (Dup)"="worker", "Mode"=enum."Worker Agent", "#Nodes"=3}, {"CSM Name (Dup)"="worker#", "Mode"=enum."Worker", "#Nodes"=3}, {"CSM Name (Dup)"="worker#", "Mode"=enum."Worker", "#Nodes"=3}, {"CSM Name (Dup)"="worker#", "Mode"=enum."Worker", "#Nodes"=3}, {"CSM Name (Dup)"="worker2", "Mode"=enum."Worker Agent", "#Nodes"=3}, {"CSM Name (Dup)"="worker2#", "Mode"=enum."Worker", "#Nodes"=3}, {"CSM Name (Dup)"="worker2#", "Mode"=enum."Worker", "#Nodes"=3}, {"CSM Name (Dup)"="worker2#", "Mode"=enum."Worker", "#Nodes"=3}] ("Module Status Array 2")
          # "Reserved constants with chain&worker nodes info"
        }
        frame Enabled {
        }
      }
      n123 = And Array Elements(Boolean array=w46) -> (logical AND=w17:bool)
      n124 = Unbundle By Name(cluster{"Mode":T1, "#Nodes":i32} {"Mode"=enum."Stand Alone", "#Nodes"=1} ("Module Status")) -> ("Mode"=w37:T1, "#Nodes"=w35:i32)
      n125 = Unbundle By Name(w39) -> ("Mode"=w36:T1, "#Nodes"=w34:i32)
      n126 = Select(t=w11, s=w17, f=w12) -> (s? t:f=w16:string)
      n127 = Select(t=w11, s=w15, f=w12) -> (s? t:f=w14:string)
      n128 = call "Package Error Info.vi"("error in"=w7, "String in"="General error") -> ("packed error info out"=w23:string, "error status"=w24:bool)  [unwired: 8 in]
      n129 = Equal?(x=w37, y=w36) -> (x = y?=w32:bool)
      n130 = Equal?(x=w35, y=w34) -> (x = y?=w33:bool)
      n131 = And(x=w32, y=w33) -> (x .and. y?=w13:bool)
      n132 = Select(t=w11, s=w13, f=w12) -> (s? t:f=w10:string)
      n133 = call-dynamic "failIf.vi"("message (\"\")"=w23, "fail"=w24, "TestCase in"=w22) -> ("error out"=w20:errorcluster, "TestCase out"=w21:refnum<class "testcase-CSMManagementAPI.lvclass">)  [unwired: 7 in]
      n134 = Compound Arithmetic op=AND(w17, w15, w13) -> (w31:bool)
      n135 = Concatenate Strings("module status failure" ("message (\"\")"), w16, w14, w10) -> (w9:string)
      n136 = call-dynamic "passIf.vi"("error in (no error)"=w20, "message (\"\")"=w9, "pass"=w31, "TestCase in"=w21) -> ("error out"=w64:errorcluster, "TestCase out"=w65:refnum<class "testcase-CSMManagementAPI.lvclass">)  [unwired: 6 in]
    }
    frame Disabled {
      # "skip test result while test is under development"
      n137 = call <vilib>:"skip.vi"("error in (no error)"=w381, "TestCase in"=w384) -> ("error out"=w383:errorcluster, "TestCase out"=w382:refnum<class "testcase-CSMManagementAPI.lvclass">)  [unwired: 8 in]
    }
  }
  "error out" <- w4
  "TestCase out" <- w2
